vi "Switch Camera.vi"(10 "New Camera":T1) -> ()   [LabVIEW 2016]
uses:
  Vision/CameraEnum.ctl
  <vilib>/Rock Robotics/Network Tables/NT Write Boolean.vi
  Robot Global Data.vi
  <vilib>/Rock Robotics/Network Tables/NT Write Number.vi
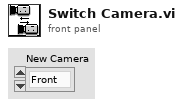
[diagram p1: front panel]
types:
  T1 = typedef "CameraEnum.ctl" = enum16{"Front", "Back"}
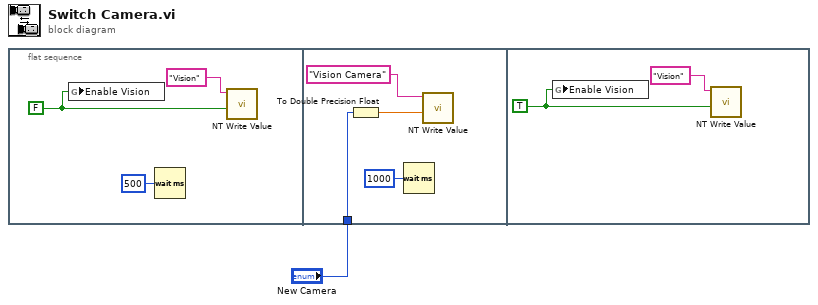
[diagram p0: block diagram]
diagram:
  n1 = flat-sequence {
    tunnel: "New Camera" -> [w5]
    frame #0 {
      w3 = FALSE ("Boolean")
      n2 = global write "Robot Global Data.vi" "Enable Vision"(w3) -> ()
      n3 = Wait (ms)(milliseconds to wait=u32 500) -> ()  [unwired: 1 out]
      n4 = call-poly <vilib>:"NT Write Value.vi"("Boolean"=w3, "Name"="Vision") -> ()  [unwired: 9 in, 1 out]
    }
    frame #1 {
      n5 = To Double Precision Float(number=w5) -> (double precision float=w7:dbl)
      n6 = Wait (ms)(milliseconds to wait=u32 1000) -> ()  [unwired: 1 out]
      n7 = call-poly <vilib>:"NT Write Value.vi"("Numeric"=w7, "Name"="Vision Camera") -> ()  [unwired: 9 in, 1 out]
    }
    frame #2 {
      w10 = TRUE ("Boolean")
      n8 = global write "Robot Global Data.vi" "Enable Vision"(w10) -> ()
      n9 = call-poly <vilib>:"NT Write Value.vi"("Boolean"=w10, "Name"="Vision") -> ()  [unwired: 9 in, 1 out]
    }
  }
